vi "Unpack for gRPC.vi"(8 "error in":errorcluster, 9 "configuration / results":enum16{"Configuration", "Results"}(ring), 10 "any":T1, 11 "measurement plugin in":refnum<class "FPT_SParam.lvclass">) -> (0 "error out":errorcluster, 2 "data value":variant, 3 "measurement plugin out":refnum<class "FPT_SParam.lvclass">)   [LabVIEW 2023, in "FPT_SParam.lvclass"]
uses:
  FPT_SParam.lvclass
  <vilib>/gRPC/LabVIEW gRPC Library/Shared/Any.ctl
  C:/Program Files/National Instruments/LabVIEW 2023/vi.lib/Plug-In SDKs/Measurements/Measurement Plugin Service/Measurement Plugin Service.lvclass
  Measurement Configuration.ctl
  Measurement Results.ctl
  a521b266-ce99-437c-923d-067dcf1e07fd.vi
  3ecd018e-d556-4cbc-bc60-c4ba57204520.vi
  <vilib>/gRPC/LabVIEW gRPC Library/Server API/Translate Protobuf Error.vi
  <vilib>/AdvancedString/1D String Array to Delimited String.vi
  <vilib>/gRPC/LabVIEW gRPC Library/Server API/Server/Get Server DLL Path.vi
  FPT_SParam.lvclass/FPT_SParam.ctl
  <vilib>/Plug-In SDKs/Measurements/Measurement Plugin Service/Measurement Plugin Service.lvclass
  <vilib>/gRPC/LabVIEW gRPC Library/grpc-lvsupport-release.lvlib
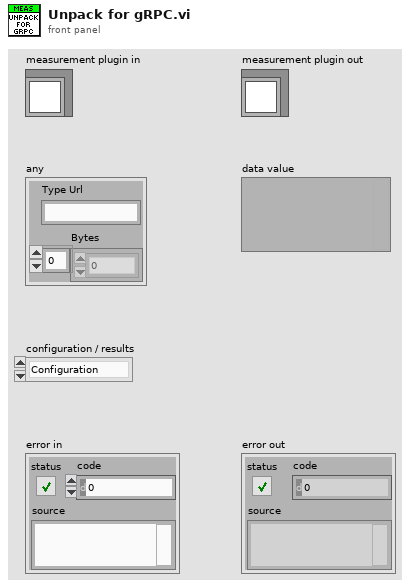
[diagram p1: front panel]
types:
  T1 = typedef "grpc-lvsupport-release.lvlib/Any.ctl" = cluster{"Type Url":string, "Bytes":u8[]}
  T2 = typedef "grpc-lvsupport-release.lvlib/grpcId.ctl" = u64
  T3 = typedef "FPT_SParam.lvclass/Measurement Configuration.ctl" = cluster{"Automation Test":bool, "Power sequencing file path":string, "RFmxVNA name":string, "vCal Name":string, "RFmxVNA Calset Enable":bool, "RFmxVNA Calset Interpolation":bool, "Calset File Path (String)":string, "RFmxVNA attenuation mode":enum32{"<None>", "s2p File"}, "RFmxVNA Port1 s2p file path (String)":string, "RFmxVNA Port1 s-parameters orientation":enum32{"Port1 Towards DUT", "Port2 Towards DUT"}, "RFmxVNA Port1 Power Compensation":bool, "RFmxVNA Port2 s2p file path (String)":string, "RFmxVNA Port2 s-parameters orientation":enum32{"Port1 Towards DUT", "Port2 Towards DUT"}, "RFmxVNA Port2 Power Compensation":bool, "Port1 Power Level (dBm)":dbl, "Port1 Test Receiver Attenuation (dB)":dbl, "Port2 Power Level (dBm)":dbl, "Port2 Test Receiver Attenuation (dB)":dbl, "IF Bandwidth (Hz)":dbl, "Action":enum32{"Calibrate", "Measure"}, "Pulse Mode Enabled":bool, "Pulse Period":dbl, "Pulse Modulator Delay":dbl, "Pulse Modulator Width":dbl, "Pulse Acquisition Auto":bool, "Pulse Acquisition Delay":dbl, "Pulse Acquisition Width":dbl, "Start Frequency (Hz)":dbl, "Stop Frequency (Hz)":dbl, "Number of Points":i32, "Measurement S-Parameters":string[], "Phase Trace Type":i32, "Magnitude Units":i32, "SnP File Path (String)":string, "Averaging Enabled":bool, "Averaging Count":u32}
  T4 = typedef "FPT_SParam.lvclass/Measurement Results.ctl" = cluster{"Status":string, "S-Param Name":string[], "S-Param Magnitude":dbl[][], "S-Param Phase":dbl[][], "VNA Status":string}
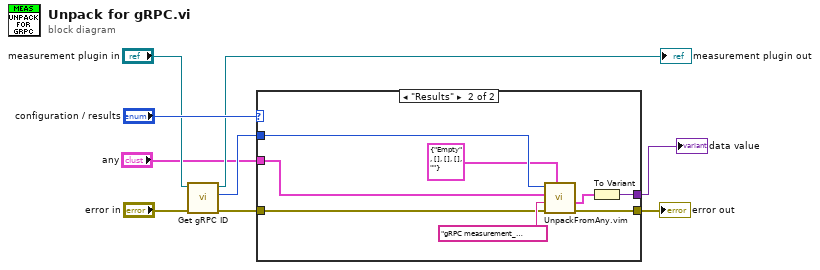
[diagram p0: block diagram]
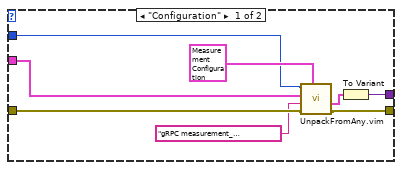
[diagram p2: hidden frame]
diagram:
  n1 = call <vilib>:"Get gRPC ID.vi"("error in"="error in", "measurement plugin service in"="measurement plugin in") -> ("error out"=w6:errorcluster, "gRPC ID"=w3:T2, "measurement plugin service out"=→"measurement plugin out":refnum<class "FPT_SParam.lvclass">)  [unwired: 7 in]
  n2 = case shown="\"Results\"" "configuration / results" {
    tunnel: w6 -> [w15 w19]
    tunnel: "any" -> [w10 w18]
    tunnel: w3 -> [w12 w22]
    tunnel: [w16 w23] -> w9
    tunnel: [w17 w25] -> w1
    frame "Configuration" {
      n3 = call "UnpackFromAny.vim"("Data Type"=T3 {"Automation Test"=FALSE, "Power sequencing file path"="Lorem ipsum dolor sit", "RFmxVNA name"="5842_0", "vCal Name"="", "RFmxVNA Calset Enable"=FALSE, "RFmxVNA Calset Interpolation"=FALSE, "Calset File Path (String)"="", "RFmxVNA attenuation mode"=enum."s2p File", "RFmxVNA Port1 s2p file path (String)"="", "RFmxVNA Port1 s-parameters orientation"=enum."Port2 Towards DUT", "RFmxVNA Port1 Power Compensation"=FALSE, "RFmxVNA Port2 s2p file path (String)"="", "RFmxVNA Port2 s-parameters orientation"=enum."Port1 Towards DUT", "RFmxVNA Port2 Power Compensation"=FALSE, "Port1 Power Level (dBm)"=0.0, "Port1 Test Receiver Attenuation (dB)"=1.0, "Port2 Power Level (dBm)"=1.0, "Port2 Test Receiver Attenuation (dB)"=0.0, "IF Bandwidth (Hz)"=100000.0, "Action"=enum."Measure", "Pulse Mode Enabled"=FALSE, "Pulse Period"=0.001, "Pulse Modulator Delay"=0.0, "Pulse Modulator Width"=0.0001, "Pulse Acquisition Auto"=FALSE, "Pulse Acquisition Delay"=2e-05, "Pulse Acquisition Width"=4.665e-05, "Start Frequency (Hz)"=4000000000.0, "Stop Frequency (Hz)"=26000000000.0, "Number of Points"=200, "Measurement S-Parameters"=["S11", "S12", "S21", "S22"], "Phase Trace Type"=0, "Magnitude Units"=0, "SnP File Path (String)"="", "Averaging Enabled"=FALSE, "Averaging Count"=0} ("Measurement Configuration"), "error in"=w15, "Message Type"="gRPC measurement_measurement configuration", "Any"=w10, "gRPCid in"=w12) -> ("error out"=w16:errorcluster, "Unpacked Value"=w14:T3)  [unwired: 4 in, 1 out]
      n4 = To Variant(anything=w14) -> (Variant=w17:variant)
    }
    frame "Results" {
      n5 = call "UnpackFromAny.vim"("Data Type"=T4 {"Status"="Empty", "S-Param Name"=[], "S-Param Magnitude"=[], "S-Param Phase"=[], "VNA Status"=""} ("Measurement Results"), "error in"=w19, "Message Type"="gRPC measurement_measurement results", "Any"=w18, "gRPCid in"=w22) -> ("error out"=w23:errorcluster, "Unpacked Value"=w24:T4)  [unwired: 4 in, 1 out]
      n6 = To Variant(anything=w24) -> (Variant=w25:variant)
    }
  }
  "error out" <- w9
  "data value" <- w1
